vi "CalculatorCode.vi"() -> ()   [LabVIEW 2015]
panel:
  out "x/y":dbl
  out "x*y":dbl
  out "x-y":dbl
  out "x+y":dbl
  in  "y":dbl
  in  "x":dbl
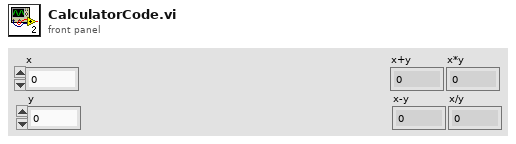
[diagram p1: front panel]
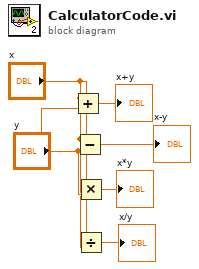
[diagram p0: block diagram]
diagram:
  n1 = Add(x="x", y="y") -> (x+y=→"x+y":dbl)
  n2 = Subtract(x="x", y="y") -> (x-y=→"x-y":dbl)
  n3 = Multiply(x="x", y="y") -> (x*y=→"x*y":dbl)
  n4 = Divide(x="x", y="x") -> (x/y=→"x/y":dbl)
